vi "manip_status_loop_maxon.vi"(8 "error in":errorcluster) -> (0 "error out":errorcluster)   [LabVIEW 2014]
doc: "The UDP protocol differs from TCP in that there is no error-checking with the packets of information that are sent, and thus no guarantee whatsoever that an intended recipient will actually receive a given piece of data.\n\nUDP does offer the ability to \"broadcast\" data across a network--simply specify an IP Address of all ones (255.255.255.255) to attempt to broadcast information network-wide. Keep in mind that routers and other network hardware will generally refuse to forward the broadcast beyond certain points, so the extent of the broadcast will in practice be limited."
uses:
  <vilib>/Platform/TimedLoop/XDataNode/timing_clust.ctl
  <vilib>/Platform/TimedLoop/XDataNode/nitl_modes.ctl
  <vilib>/Platform/TimedLoop/XDataNode/wakeup.ctl
  <vilib>/Platform/TimedLoop/XDataNode/XDataNode.xnode
  <vilib>/Platform/TimedLoop/XDataNode/XDNodeRunTimeDep.lvlib
panel:
  out "Status and error":u32[][](array[numeric]) format="%x"
  out "Motion":sgl[][](array[numeric]) format="%.3f"
  out "length":i32
  out "Rx packets":i32
  in  "receiver port":u16=61559
  # "This loops reading back status from interface for the Maxon manipulator."
  # "Status"
  # "Error"
  # "Position"
  # "Velocity"
  # "Current"
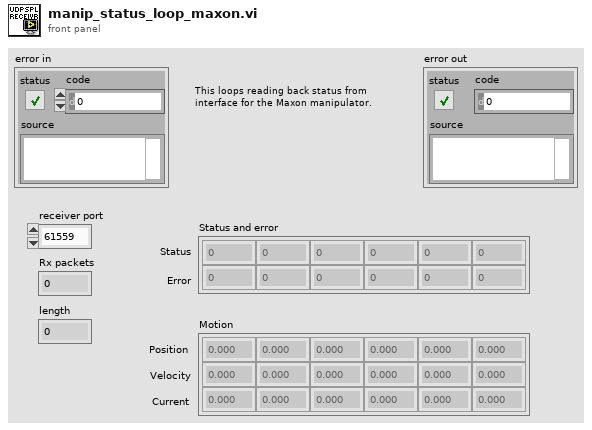
[diagram p1: front panel]
types:
  T1 = typedef "XDNodeRunTimeDep.lvlib/timing_clust.ctl" = cluster{"Expected End [f-1]":u64, "Actual End [f-1]":u64, "Finished Late? [f-1]":bool, "Expected End [i-1]":u64, "Actual End [i-1]":u64, "Finished Late? [i-1]":bool, "Expected Start [i]":u64, "Actual Start [i]":u64, "Expected Start [f]":u64, "Actual Start [f]":u64, "Source Name":string, "Structure Name":string, "Period":i64, "Deadline":i64, "Offset":i64, "Start":i64, "Priority":i32, "Timeout":i32, "Mode":T2, "Wakeup Reason":T3, "Error":errorcluster, "Source Type":string, "Secondary Source Type":string, "Global End Time":u64, "Global Start Time":u64, "Frame Duration":u64, "Iteration Duration":u64, "Assigned CPU":i32, "I/O Scan Engine Mode":u32}
  T2 = typedef "XDNodeRunTimeDep.lvlib/nitl_modes.ctl" = enum32{"No Change", "Process missed periods, maintain original phase", "Discard missed periods, maintain original phase", "Process missed periods, ignore original phase", "Discard missed periods, ignore original phase"}
  T3 = typedef "XDNodeRunTimeDep.lvlib/wakeup.ctl" = enum32{"Normal", "Aborted", "Asynchronous wakeup", "Timing source error", "Timed loop error", "Timeout"}
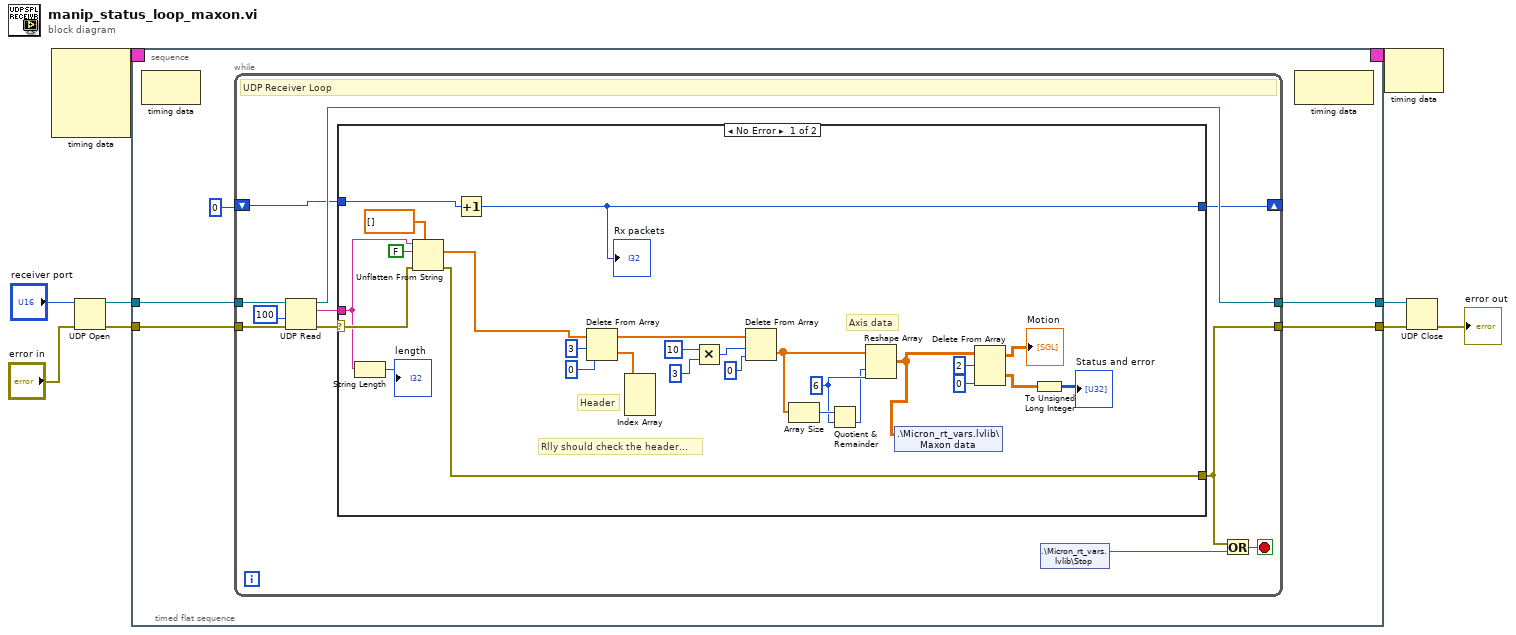
[diagram p0: block diagram]
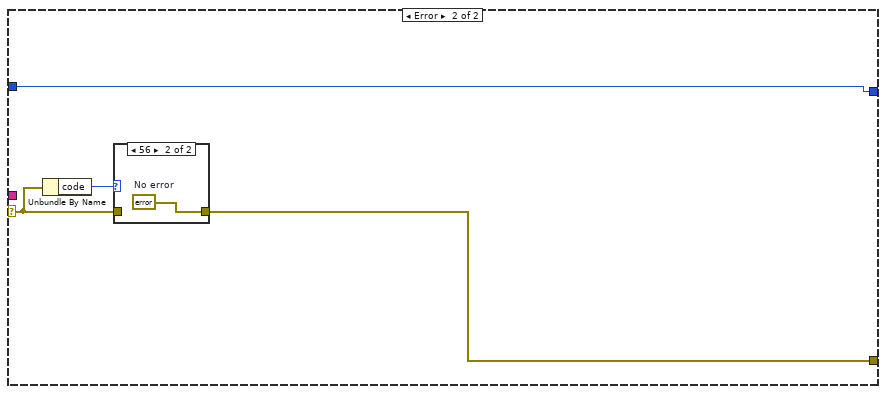
[diagram p2: hidden frame]
diagram:
  n1 = node-c288() -> (w2:T1)  [unwired: 4 in]
  n2 = UDP Open(8:"error in", 11:"receiver port") -> (port=w6:refnum<k16>, 0:w7:errorcluster)  [unwired: 3 in, 1 out]
  n3 = timed-sequence {
    timing: w2 -> [_]
    timing-out: [_] -> w1
    tunnel: [w13] -> w9
    tunnel: [w12] -> w8
    tunnel: w7 -> [w11]
    tunnel: w6 -> [w10]
    n4 = timed-flat-sequence {
      tunnel: [w18] -> w13
      tunnel: [w17] -> w12
      tunnel: w11 -> [w16]
      tunnel: w10 -> [w15]
      n5 = node-c288() -> ()  [unwired: 1 in, 1 out]
      n6 = while {
        tunnel: w15 -> [w29]
        tunnel: [w22] -> w18
        tunnel: w16 -> [w27]
        tunnel: [w23] -> w17
        shift-right: [w20] -> _
        shift-left: 0 -> [w21]
        stop <- w28 stop-if-true
        # "UDP Receiver Loop"
        n7 = UDP Read(connection ID=w29, timeout ms (25000)=100, 8:w27) -> (data out=w25:string, error out=w24:errorcluster, 3:w22:refnum<k16>)  [unwired: 3 out]
        n8 = case shown="No Error" w24 {
          selector: w24 -> [w55 w59]
          tunnel: w25 -> [w53 _]
          tunnel: [w38 w58] -> w23
          tunnel: w21 -> [w54 w57]
          tunnel: [w51 w57] -> w20
          frame No Error {
            w37 = 6 ("dimension size")
            # "Rlly should check the header..."
            # "Axis data"
            # "Header"
            # "Sender sent data. Update the chart value."
            n9 = String Length(string=w53) -> (length=→"length":i32)
            n10 = Unflatten From String(type=sgl[] [], binary string=w53, data includes array or string size? (T)=FALSE, error in (no error)=w55) -> (value=w49:sgl[], error out=w38:errorcluster)  [unwired: 1 in, 1 out]
            n11 = Increment(x=w54) -> (x+1=w51:i32)
            "Rx packets" <- w51
            n12 = Delete From Array(array=w49, length=3, index=0) -> (deleted portion=w46:sgl[], array with subset deleted=w45:sgl[])
            n13 = Index Array(array=w46) -> ()  [unwired: 3 in, 3 out]
            n14 = Multiply(x=10, y=3) -> (x*y=w44:i32)
            n15 = Delete From Array(array=w45, length=w44, index=0) -> (deleted portion=w40:sgl[])  [unwired: 1 out]
            n16 = Array Size(array=w40) -> (size(s)=w39:i32)
            n17 = Quotient & Remainder(x=w39, y=w37) -> (floor(x/y)=w36:i32)  [unwired: 1 out]
            n18 = Reshape Array(w40, w36, w37) -> (w35:sgl[][])
            n19 = shared-variable ".\\Micron_rt_vars.lvlib\\Maxon data"(w35) -> ()  [unwired: 1 in, 1 out]
            n20 = Delete From Array(array=w35, length=2, index (row)=0) -> (deleted portion=w31:sgl[][], array with subset deleted=→"Motion":sgl[][])  [unwired: 1 in]
            n21 = To Unsigned Long Integer(number=w31) -> (unsigned 32bit integer=→"Status and error":u32[][])
          }
          frame Error {
            # "Sender did not send data. Ignore timeout error and keep waiting."
            n22 = Unbundle By Name(w59) -> ("code"=w60:i32)
            n23 = case shown="56" w60 {
              tunnel: w59 -> [w61 _]
              tunnel: [w61 w62] -> w58
              frame Default {
              }
              frame 56 {
                w62 = errorcluster {"status"=FALSE, "code"=0, "source"=""}  # No error
              }
            }
          }
        }
        n24 = shared-variable ".\\Micron_rt_vars.lvlib\\Stop"() -> (w19:bool)  [unwired: 2 out]
        n25 = Or(x=w23, y=w19) -> (x .or. y?=w28:bool)
      }
      n26 = node-c288() -> ()  [unwired: 1 in, 1 out]
    }
  }
  n27 = node-c288(w1) -> ()  [unwired: 1 out]
  n28 = UDP Close(connection ID=w9, 8:w8) -> (error out=→"error out":errorcluster)  [unwired: 1 out]
